vi "Clamp Wrapper.vi"(0 "In":bool, 1 "Out":bool, 2 "Iterations":i32=1) -> ()   [LabVIEW 2014]
uses:
  Precreated VIs/Robot Global Data.vi
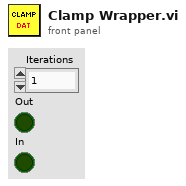
[diagram p1: front panel]
types:
  T1 = cluster{"Limit Switches":cluster{"Lift":cluster{"Top":bool, "High":bool, "Mid":bool, "Low":bool, "Bot":bool}, "Clamp":cluster{"Widest":bool, "Shortest":bool, "Tote 1":bool, "Tote 2":bool}, "Tote Detected":bool}, "Ultrasonic":dbl, "Beam Breaker Clamp":bool, "Lift Encoder":dbl}
  T2 = cluster{"Manual Lift":dbl, "Manual Clamp":dbl, "Auto Lift Up":bool, "Auto Lift Down":bool, "Auto Clamp In":bool, "Auto Clamp Out":bool, "Clamp Latch":bool, "Lift Stop":bool, "Clamp Stop":bool}
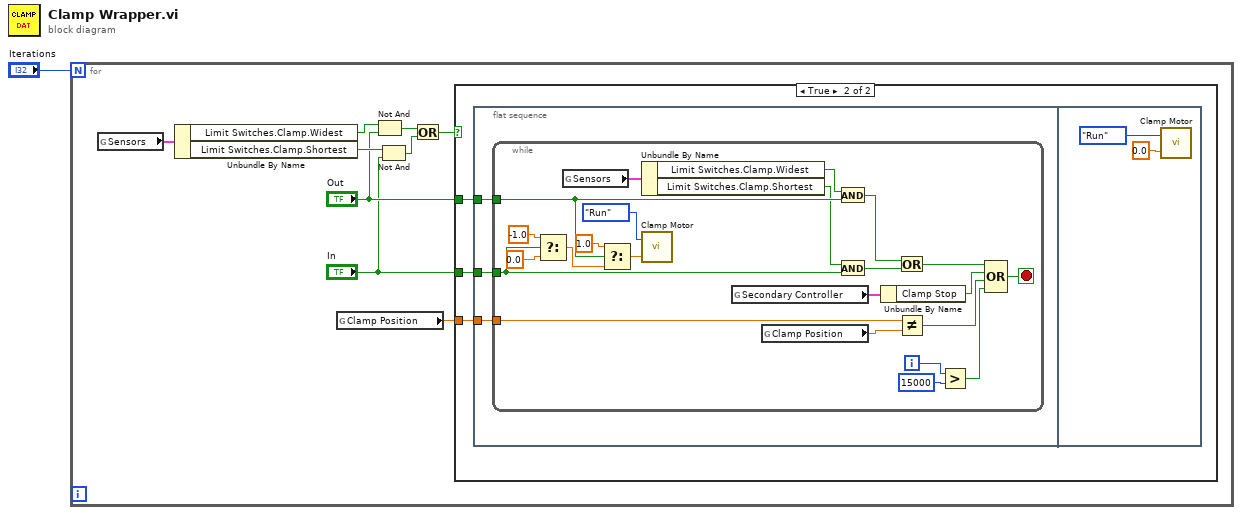
[diagram p0: block diagram]
diagram:
  n1 = for {
    N: "Iterations" -> [_]
    n2 = global read "Robot Global Data.vi" "Sensors"() -> (w8:T1)
    n3 = Unbundle By Name(w8) -> ("Limit Switches.Clamp.Widest"=w5:bool, "Limit Switches.Clamp.Shortest"=w4:bool)
    n4 = global read "Robot Global Data.vi" "Clamp Position"() -> (w9:dbl)
    n5 = Not And(1:"Out", 2:w5) -> (0:w7:bool)
    n6 = Not And(1:"In", 2:w4) -> (0:w6:bool)
    n7 = Or(x=w7, y=w6) -> (x .or. y?=w10:bool)
    n8 = case shown="True" w10 {
      tunnel: "Out" -> [_ w13]
      tunnel: "In" -> [_ w12]
      tunnel: w9 -> [_ w11]
      frame False {
      }
      frame True {
        n9 = flat-sequence {
          tunnel: w13 -> [w16]
          tunnel: w12 -> [w15]
          tunnel: w11 -> [w14]
          frame #0 {
            n10 = while {
              tunnel: w16 -> [w22]
              tunnel: w15 -> [w21]
              tunnel: w14 -> [w36]
              i -> [w28]
              stop <- w25 stop-if-true
              n11 = Select(t=-1.0, s=w21, f=0.0) -> (s? t:f=w38:dbl)
              n12 = global read "Robot Global Data.vi" "Sensors"() -> (w24:T1)
              n13 = Select(t=1.0, s=w22, f=w38) -> (s? t:f=w32:dbl)
              n14 = Unbundle By Name(w24) -> ("Limit Switches.Clamp.Widest"=w23:bool, "Limit Switches.Clamp.Shortest"=w20:bool)
              n15 = call "Clamp Motor.vi"("Speed"=w32, "Mode"=enum8{"Start", "Run", "Finish"}."Run") -> ()  [unwired: 1 in]
              n16 = global read "Robot Global Data.vi" "Secondary Controller"() -> (w31:T2)
              n17 = global read "Robot Global Data.vi" "Clamp Position"() -> (w37:dbl)
              n18 = And(x=w23, y=w22) -> (x .and. y?=w19:bool)
              n19 = And(x=w20, y=w21) -> (x .and. y?=w18:bool)
              n20 = Unbundle By Name(w31) -> ("Clamp Stop"=w30:bool)
              n21 = Or(x=w19, y=w18) -> (x .or. y?=w17:bool)
              n22 = Not Equal?(x=w36, y=w37) -> (x != y?=w29:bool)
              n23 = Greater?(x=w28, y=15000) -> (0:w26:bool)
              n24 = Compound Arithmetic op=OR(w17, w30, w29, w26) -> (w25:bool)
            }
          }
          frame #1 {
            n25 = call "Clamp Motor.vi"("Speed"=0.0, "Mode"=enum8{"Start", "Run", "Finish"}."Run") -> ()  [unwired: 1 in]
          }
        }
      }
    }
  }
